vi "Flush Data to Log File.vi"(8 "error in (no error)":errorcluster, 10 "Data Queue":refnum<queue>, 11 "Logging Configuration":T1={"Log Directory Path"=path "", "Log File Path"=path "", "Log File Prefix"="", "Log File Extension"="", "File Delimiter"=",", "Header Info"=[], "Channels"=[], "Log Instrument Runs"=FALSE}) -> (0 "error out":errorcluster)   [LabVIEW 2020, in "Deep Reaction Optimizer Control Panel.lvlib" / "Logging.lvlib"]
doc: "Flush the data queue of any pending data and write it to the log file. Close the TDMS file reference."
uses:
  Logging.lvlib
  Instrument Manager/Instrument State.ctl
  <vilib>/addons/zeromq/zmq_context.lvclass
  <vilib>/addons/zeromq/zmq_socket.lvclass
  Logging Configuration.ctl
  <vilib>/Utility/file.llb/Write Delimited Spreadsheet (string).vi
  Instrument Manager/Instrument Manager.lvlib
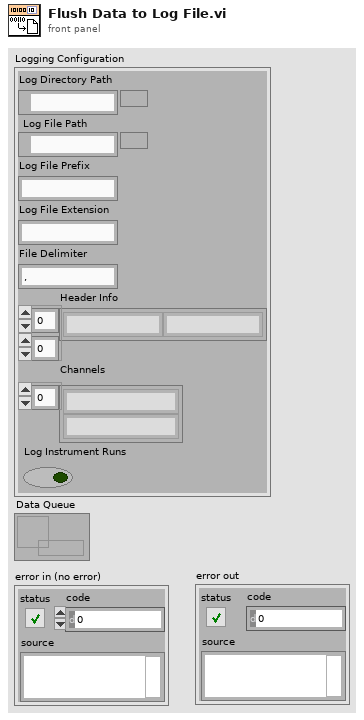
[diagram p1: front panel]
types:
  T1 = typedef "Deep Reaction Optimizer Control Panel.lvlib/Logging.lvlib/Logging Configuration.ctl" = cluster{"Log Directory Path":path, "Log File Path":path, "Log File Prefix":string, "Log File Extension":string, "File Delimiter":string, "Header Info":string[][], "Channels":string[], "Log Instrument Runs":bool}
  T2 = typedef "Deep Reaction Optimizer Control Panel.lvlib/Instrument Manager.lvlib/Instrument State.ctl" = cluster{"Context":refnum<class "zmq_context.lvclass">, "Socket":refnum<class "zmq_socket.lvclass">, "Running Since":timestamp, "New Parameters (values)":cluster{"Time Stamp":timestamp, "Name":string[], "Value":dbl[]}, "Optimizer Path":path, "Running":bool, "Response Counter":u8, "Response Timeout (ms)":u32, "Response Retries":u32, "Endpoint":string, "Starting up?":bool, "New Parameters (percents)":cluster{"Time Stamp":timestamp, "Name":string[], "Value":dbl[]}, "Flow Rate Constant":dbl, "Yield":dbl}
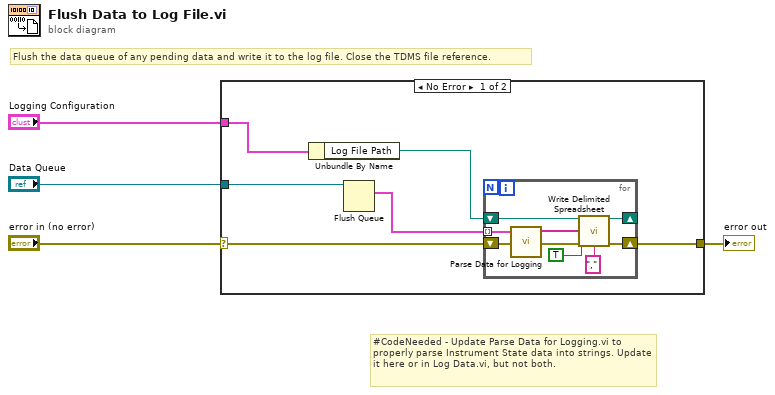
[diagram p0: block diagram]
diagram:
  # "#CodeNeeded - Update Parse Data for Logging.vi to properly parse Instrument State data into strings. Update it here or in Log Data.vi, but not both."
  # "Flush the data queue of any pending data and write it to the log file. Close the TDMS file reference."
  n1 = case shown="No Error" "error in (no error)" {
    selector: "error in (no error)" -> [w6 w19]
    tunnel: "Data Queue" -> [w8 _]
    tunnel: "Logging Configuration" -> [w7 _]
    tunnel: [w5 w19] -> w2
    frame No Error {
      n2 = Unbundle By Name(w7) -> ("Log File Path"=w9:path)
      n3 = Flush Queue(queue=w8) -> (remaining elements=w10:T2[])  [unwired: 1 in, 2 out]
      n4 = for {
        shift-right: [w16] -> _
        shift-left: w9 -> [w17]
        shift-right: [w18] -> w5
        shift-left: w6 -> [w13]
        tunnel: w10 -> [w14] mode=indexing
        n5 = call "Parse Data for Logging.vi"("Instrument State"=w14) -> ("Array"=w12:string[])  [unwired: 10 in]
        n6 = call-poly <vilib>:"Write Delimited Spreadsheet.vi"("file path (dialog if empty)"=w17, "1D data"=w12, "append to file? (new file:F)"=TRUE, "error in (no error)"=w13, "delimiter (\\t)"="," ("delimiter (\\t)")) -> ("new file path (Not A Path if cancelled)"=w16:path, "error out"=w18:errorcluster)  [unwired: 9 in]
      }
    }
    frame Error {
    }
  }
  "error out" <- w2
